vi "Load FP Object Configuration.vi"(7 "Default Control Behavior":T4, 8 "High Level Config Settings in":T3={"Default Refresh Rate (ms)"=500, "Show Border"=FALSE, "Periodic Decoration Data"=FALSE, "Synchronous Requests"=FALSE, "Reduce Sent Data"=FALSE, "Recommended Control Settings"=FALSE}, 10 "DataRef":refnum<data-value>, 11 "Config Option":T2) -> (0 "High Level Config Settings out":T3, 1 "Indicators":T1[](array[typedef]), 2 "Controls":T1[](array[typedef]), 3 "Show Dialog":bool)   [LabVIEW 2017, in "Front Panel Publisher.lvlib" / "Web Front Panel.lvclass"]
uses:
  Web Front Panel.lvclass
  Controls/FP Object Configuration.ctl
  Controls/High Level Config Settings.ctl
  Controls/Cluster - Default Control Behavior.ctl
  Protected/Object Attributes.ctl
  Front Panel Objects/Object_class/Object.lvclass
  Common/Enum - Config Option.ctl
  Controls/Enum - Control Display Mode.ctl
  Front Panel Objects/Control_class/Control.lvclass
  Controls/All Config Settings.ctl
  <userlib>/_OpenG.lib/file/file.llb/Strip Path Extension - String__ogtk.vi
  Front Panel Publisher.lvlib
  Front Panel Manager_class/Front Panel Manager.lvclass
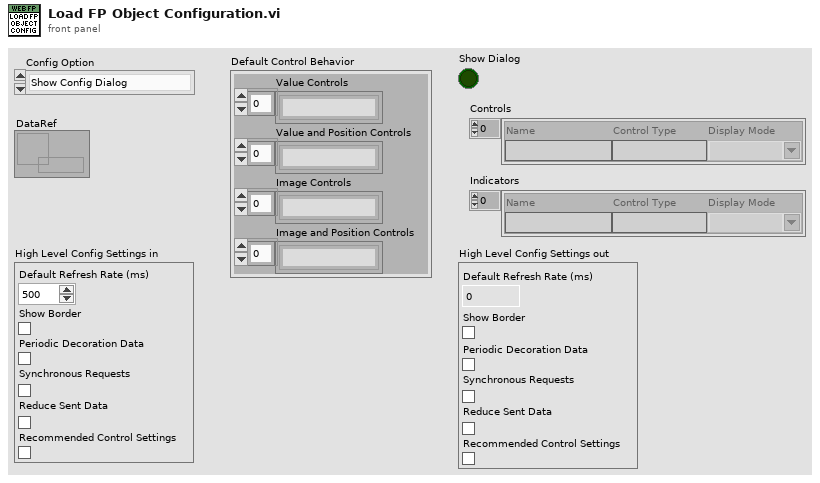
[diagram p1: front panel]
types:
  T1 = typedef "Front Panel Publisher.lvlib/Web Front Panel.lvclass/FP Object Configuration.ctl" = cluster{"Name":string, "Control Type":string, "Display Mode":string}
  T2 = typedef "Front Panel Publisher.lvlib/Enum - Config Option.ctl" = enum16{"Show Config Dialog", "Don't Show Config Dialog", "Load Config File then Show Dialog", "Load Config File No Dialog"}
  T3 = typedef "Front Panel Publisher.lvlib/Web Front Panel.lvclass/High Level Config Settings.ctl" = cluster{"Default Refresh Rate (ms)":i32, "Show Border":bool, "Periodic Decoration Data":bool, "Synchronous Requests":bool, "Reduce Sent Data":bool, "Recommended Control Settings":bool}
  T4 = typedef "Front Panel Publisher.lvlib/Web Front Panel.lvclass/Cluster - Default Control Behavior.ctl" = cluster{"Value Controls":string[], "Value and Position Controls":string[], "Image Controls":string[], "Image and Position Controls":string[]}
  T5 = typedef "Front Panel Publisher.lvlib/Web Front Panel.lvclass/Object Attributes.ctl" = cluster{"VI Identifier":string, "VI Reference":refnum<vi>, "Controls":refnum<class "Object.lvclass">[], "Indicators":refnum<class "Object.lvclass">[], "Decorations":refnum<class "Object.lvclass">[], "VR With Previous Get":refnum<data-value>, "VR With Ring Images":refnum<data-value>}
  T6 = typedef "Front Panel Publisher.lvlib/Web Front Panel.lvclass/Enum - Control Display Mode.ctl" = enum16{"Value Only", "Value and Visibility", "Boolean Value Only", "Boolean Value and Visibility", "Control is Image", "Image and Visibility"}
  T7 = typedef "Front Panel Publisher.lvlib/Web Front Panel.lvclass/All Config Settings.ctl" = cluster{"Objects Configurations":T1[], "High Level Config Settings":T3}
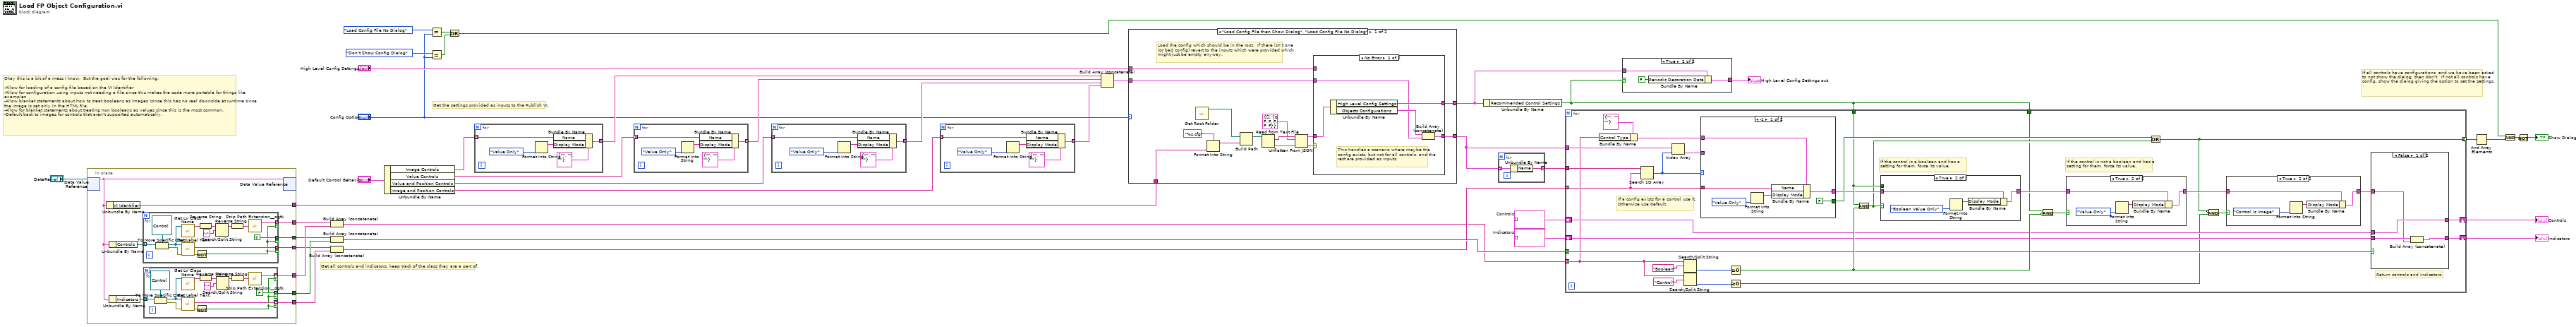
[diagram p0: block diagram]
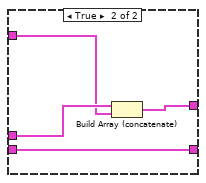
[diagram p3: hidden frame]
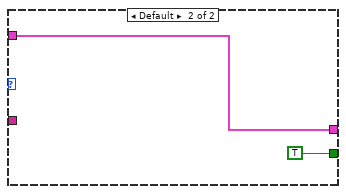
[diagram p6: hidden frame]
diagram:
  w10 = T1[] []  # Indicators
  w11 = T1[] []  # Controls
  # "If all controls have configurations, and we have been asked to not show the dialog, then don't.  If not all controls have config, show the dialog giving the option to set the settings."
  # "Get the settings provided as inputs to the Publish VI."
  # "Get all controls and indicators, keep track of the class they are a part of."
  # "Okay this is a bit of a mess I know.  But the goal was for the following:\n\n-Allow for loading of a config file based on the VI Identifier\n-Allow for configuration using inputs not needing a file since this makes the code more portable for things like examples\n-Allow blanket statements about how to treat booleans as images (since this has no real downside at runtime since the image is set only in the HTML file.\n-Allow for blanket statements about treating non booleans as values since this is the most common.\n-Default back to images for controls that aren't supported automatically."
  n1 = in-place {
    in-place-border: [w49] -> w34
    in-place-border: [w48] -> w39
    in-place-border: [w47] -> w33
    in-place-border: [w45] -> w38
    in-place-border: [w44] -> w37
    in-place-border: [w43] -> w36
    in-place-border: [w42] -> w35
    n2 = in-place-dvr #1("DataRef") -> (w46:T5)  [unwired: 1 out]
    n3 = Unbundle By Name(w46) -> ("VI Identifier"=w48:string)
    n4 = Unbundle By Name(w46) -> ("Controls"=w51:refnum<class "Object.lvclass">[])
    n5 = Unbundle By Name(w46) -> ("Indicators"=w50:refnum<class "Object.lvclass">[])
    n6 = for {
      tunnel: w51 -> [w79] mode=indexing
      tunnel: [w76] -> w49 mode=indexing if=w72
      tunnel: [w66] -> w45 mode=indexing if=w72
      tunnel: [TRUE] -> w43 mode=indexing if=w72
      n7 = To More Specific Class(target class=refnum<class "Control.lvclass"> refnum ("FrontPanelPublisher.lvlib:Control"), reference=w79) -> (specific class reference=w74:refnum<class "Control.lvclass">, error out=w77:errorcluster)  [unwired: 1 in]
      n8 = call <vilib>:"Get LV Class Name.vi"("object"=w74) -> ("class name"=w67:string)  [unwired: 9 in, 1 out]
      n9 = call-dynamic "Get Label Text.vi"("error in (no error)"=w77, "Control In"=w74) -> ("error out"=w75:errorcluster, "Text"=w76:string)  [unwired: 7 in, 1 out]
      n10 = Not(x=w75) -> (.not. x?=w72:bool)
      n11 = Reverse String(1:w67) -> (0:w69:string)
      n12 = Search/Split String(string=w69, search string/char (-)=":") -> (substring before match=w70:string)  [unwired: 1 in, 2 out]
      n13 = Reverse String(1:w70) -> (0:w71:string)
      n14 = call-poly <userlib>:"Strip Path Extension__ogtk.vi"("path"=w71) -> ("root"=w66:string)  [unwired: 1 out]
    }
    n15 = for {
      tunnel: w50 -> [w65] mode=indexing
      tunnel: [w62] -> w47 mode=indexing if=w58
      tunnel: [w54] -> w44 mode=indexing if=w58
      tunnel: [FALSE] -> w42 mode=indexing if=w58
      n16 = To More Specific Class(target class=refnum<class "Control.lvclass"> refnum ("FrontPanelPublisher.lvlib:Control"), reference=w65) -> (specific class reference=w60:refnum<class "Control.lvclass">, error out=w63:errorcluster)  [unwired: 1 in]
      n17 = call <vilib>:"Get LV Class Name.vi"("object"=w60) -> ("class name"=w53:string)  [unwired: 9 in, 1 out]
      n18 = call-dynamic "Get Label Text.vi"("error in (no error)"=w63, "Control In"=w60) -> ("error out"=w61:errorcluster, "Text"=w62:string)  [unwired: 7 in, 1 out]
      n19 = Not(x=w61) -> (.not. x?=w58:bool)
      n20 = Reverse String(1:w53) -> (0:w56:string)
      n21 = Search/Split String(string=w56, search string/char (-)=":") -> (substring before match=w55:string)  [unwired: 1 in, 2 out]
      n22 = Reverse String(1:w55) -> (0:w52:string)
      n23 = call-poly <userlib>:"Strip Path Extension__ogtk.vi"("path"=w52) -> ("root"=w54:string)  [unwired: 1 out]
    }
    n24 = in-place-dvr #1(w46) -> ()  [unwired: 2 out]
  }
  n25 = Build Array (concatenate)(w38, w37) -> (w5:string[])
  n26 = Build Array (concatenate)(w36, w35) -> (w13:bool[])
  n27 = Build Array (concatenate)(w34, w33) -> (w6:string[])
  n28 = Unbundle By Name("Default Control Behavior") -> ("Image Controls"=w31:string[], "Value Controls"=w30:string[], "Value and Position Controls"=w29:string[], "Image and Position Controls"=w4:string[])
  n29 = Equal?(x=Enum_-_Config_Option."Load Config File No Dialog", y="Config Option") -> (x = y?=w17:bool)
  n30 = Equal?(x=Enum_-_Config_Option."Don't Show Config Dialog", y="Config Option") -> (x = y?=w16:bool)
  n31 = Or(x=w17, y=w16) -> (x .or. y?=w15:bool)
  n32 = for {
    tunnel: w31 -> [w83] mode=indexing
    tunnel: [w82] -> w26 mode=indexing
    n33 = Format Into String(Enum_-_Control_Display_Mode."Value Only" ("Enum")) -> (resulting string=w80:string)  [unwired: 3 in, 1 out]
    n34 = Bundle By Name(cluster=T1 {"Name"="", "Control Type"="", "Display Mode"=""} ("FP Object Configuration"), "Name"=w83, "Display Mode"=w80) -> (w82:T1)
  }
  n35 = for {
    tunnel: w30 -> [w88] mode=indexing
    tunnel: [w87] -> w27 mode=indexing
    n36 = Format Into String(Enum_-_Control_Display_Mode."Value Only" ("Enum")) -> (resulting string=w85:string)  [unwired: 3 in, 1 out]
    n37 = Bundle By Name(cluster=T1 {"Name"="", "Control Type"="", "Display Mode"=""} ("FP Object Configuration"), "Name"=w88, "Display Mode"=w85) -> (w87:T1)
  }
  n38 = for {
    tunnel: w29 -> [w93] mode=indexing
    tunnel: [w92] -> w28 mode=indexing
    n39 = Format Into String(Enum_-_Control_Display_Mode."Value Only" ("Enum")) -> (resulting string=w90:string)  [unwired: 3 in, 1 out]
    n40 = Bundle By Name(cluster=T1 {"Name"="", "Control Type"="", "Display Mode"=""} ("FP Object Configuration"), "Name"=w93, "Display Mode"=w90) -> (w92:T1)
  }
  n41 = for {
    tunnel: w4 -> [w98] mode=indexing
    tunnel: [w97] -> w3 mode=indexing
    n42 = Format Into String(Enum_-_Control_Display_Mode."Value Only" ("Enum")) -> (resulting string=w95:string)  [unwired: 3 in, 1 out]
    n43 = Bundle By Name(cluster=T1 {"Name"="", "Control Type"="", "Display Mode"=""} ("FP Object Configuration"), "Name"=w98, "Display Mode"=w95) -> (w97:T1)
  }
  n44 = Build Array (concatenate)(w26, w27, w28, w3) -> (w25:T1[])
  n45 = case shown="\"Load Config File then Show Dialog\", \"Load Config File No Dialog\"" "Config Option" {
    tunnel: [w108 w122] -> w24
    tunnel: [w106 w121] -> w9
    tunnel: w39 -> [w102 _]
    tunnel: "High Level Config Settings in" -> [w101 w121]
    tunnel: w25 -> [w100 w122]
    frame "Load Config File then Show Dialog", "Load Config File No Dialog" {
      # "Load the config which should be in the root.  If there isn't one (or bad config) revert to the inputs which were provided which might just be empty anyway."
      n46 = call "Get Root Folder.vi"() -> ("Root folder"=w103:path)  [unwired: 11 in]
      n47 = Format Into String(format string="%s.cfg", w102) -> (resulting string=w104:string)  [unwired: 2 in, 1 out]
      n48 = Build Path(base path=w103, name or relative path=w104) -> (appended path=w105:path)
      n49 = Read from Text File(file (use dialog)=w105) -> (text=w112:string, error out=w111:errorcluster)  [unwired: 3 in, 2 out]
      n50 = Unflatten From JSON(JSON string=w112, type and defaults=T7 {"Objects Configurations"=[], "High Level Config Settings"={"Default Refresh Rate (ms)"=0, "Show Border"=FALSE, "Periodic Decoration Data"=FALSE, "Synchronous Requests"=FALSE, "Reduce Sent Data"=FALSE, "Recommended Control Settings"=FALSE}} ("output cluster"), error in (no error)=w111) -> (value=w110:T7, error out=w109:errorcluster)  [unwired: 4 in]
      n51 = case shown="No Error" w109 {
        tunnel: w110 -> [w118 _]
        tunnel: [w114 w119] -> w108
        tunnel: [w116 w120] -> w106
        tunnel: w101 -> [_ w120]
        tunnel: w100 -> [w115 w119]
        frame No Error {
          # "This handles a scenario where maybe the config exists, but not for all controls, and the rest are provided as inputs."
          n52 = Unbundle By Name(w118) -> ("High Level Config Settings"=w116:T3, "Objects Configurations"=w117:T1[])
          n53 = Build Array (concatenate)(w117, w115) -> (w114:T1[])
        }
        frame Error {
        }
      }
    }
    frame "Show Config Dialog", "Don't Show Config Dialog", Default {
    }
  }
  n54 = Unbundle By Name(w9) -> ("Recommended Control Settings"=w1:bool)
  n55 = for {
    tunnel: w24 -> [w123] mode=indexing
    tunnel: [w124] -> w23 mode=indexing
    n56 = Unbundle By Name(w123) -> ("Name"=w124:string)
  }
  n57 = for {
    tunnel: w6 -> [w150] mode=indexing
    tunnel: w23 -> [w154]
    tunnel: w24 -> [w153]
    tunnel: [w125] -> w41 mode=indexing
    tunnel: w13 -> [w141] mode=indexing
    tunnel: w5 -> [w128] mode=indexing
    shift-right: [w138] -> w8
    shift-left: w11 -> [w139]
    shift-right: [w137] -> w7
    shift-left: w10 -> [w140]
    tunnel: w1 -> [w143]
    tunnel: w1 -> [w148]
    # "Return controls and indicators."
    # "If the control is not a boolean and has a setting for them, force its value."
    # "If the control is a boolean and has a setting for them, force its value."
    # "If a config exists for a control use it.  Otherwise use default."
    n58 = Bundle By Name(cluster=T1 {"Name"="", "Control Type"="", "Display Mode"=""} ("FP Object Configuration"), "Control Type"=w128) -> (w132:T1)
    n59 = Search 1D Array(1D array=w154, element=w150) -> (index of element=w136:i32)  [unwired: 1 in]
    n60 = Index Array(array=w153, index=w136) -> (element=w152:T1)
    n61 = Search/Split String(string=w128, search string/char (-)="Boolean") -> (offset of match=w149:i32)  [unwired: 1 in, 2 out]
    n62 = Search/Split String(string=w128, search string/char (-)="Control") -> (offset of match=w131:i32)  [unwired: 1 in, 2 out]
    n63 = case shown="-1" w136 {
      tunnel: w152 -> [_ w184]
      tunnel: [w183 w184] -> w147
      tunnel: w150 -> [w182 _]
      tunnel: [FALSE TRUE] -> w151
      tunnel: w132 -> [w178 _]
      frame -1 {
        n64 = Format Into String(Enum_-_Control_Display_Mode."Value Only" ("Enum")) -> (resulting string=w179:string)  [unwired: 3 in, 1 out]
        n65 = Bundle By Name(cluster=w178, "Name"=w182, "Display Mode"=w179) -> (w183:T1)
      }
      frame Default {
      }
    }
    n66 = Greater Or Equal To 0?(x=w149) -> (x >= 0?=w144:bool)
    n67 = Greater Or Equal To 0?(x=w131) -> (x >= 0?=w127:bool)
    n68 = And(x=w148, y=w144) -> (x .and. y?=w146:bool)
    n69 = case shown="True" w146 {
      tunnel: w148 -> [_ _]
      tunnel: w147 -> [w173 w177]
      tunnel: [w173 w176] -> w145
      frame False {
      }
      frame True {
        n70 = Format Into String(Enum_-_Control_Display_Mode."Boolean Value Only" ("Enum")) -> (resulting string=w174:string)  [unwired: 3 in, 1 out]
        n71 = Bundle By Name(cluster=w177, "Display Mode"=w174) -> (w176:T1)
      }
    }
    n72 = Compound Arithmetic op=AND(w143, invert w144) -> (w142:bool)
    n73 = case shown="True" w142 {
      tunnel: w145 -> [w168 w172]
      tunnel: [w168 w171] -> w135
      frame False {
      }
      frame True {
        n74 = Format Into String(Enum_-_Control_Display_Mode."Value Only" ("Enum")) -> (resulting string=w169:string)  [unwired: 3 in, 1 out]
        n75 = Bundle By Name(cluster=w172, "Display Mode"=w169) -> (w171:T1)
      }
    }
    n76 = Or(x=w151, y=w146) -> (x .or. y?=w125:bool)
    n77 = Compound Arithmetic op=AND(invert w125, w127) -> (w126:bool)
    n78 = case shown="True" w126 {
      tunnel: w135 -> [w155 w159]
      tunnel: [w155 w158] -> w134
      frame False {
      }
      frame True {
        n79 = Format Into String(Enum_-_Control_Display_Mode."Control is Image" ("Enum")) -> (resulting string=w156:string)  [unwired: 3 in, 1 out]
        n80 = Bundle By Name(cluster=w159, "Display Mode"=w156) -> (w158:T1)
      }
    }
    n81 = case shown="False" w141 {
      tunnel: w134 -> [w160 w165]
      tunnel: w140 -> [w162 w164]
      tunnel: w139 -> [w163 w167]
      tunnel: [w163 w166] -> w138
      tunnel: [w161 w164] -> w137
      frame False {
        n82 = Build Array (concatenate)(w162, w160) -> (w161:T1[])
      }
      frame True {
        n83 = Build Array (concatenate)(w167, w165) -> (w166:T1[])
      }
    }
  }
  "Controls" <- w8
  "Indicators" <- w7
  n84 = case shown="True" w1 {
    tunnel: w9 -> [w186 w189]
    tunnel: [w186 w188] -> w2
    frame False {
    }
    frame True {
      n85 = Bundle By Name(cluster=w189, "Periodic Decoration Data"=FALSE) -> (w188:T3)
    }
  }
  "High Level Config Settings out" <- w2
  n86 = And Array Elements(Boolean array=w41) -> (logical AND=w22:bool)
  n87 = And(x=w15, y=w22) -> (x .and. y?=w21:bool)
  n88 = Not(x=w21) -> (.not. x?=→"Show Dialog":bool)
